vi "PM5000_Harmonics_Results.vi"(8 "error in":errorcluster, 11 "Network Path":string="172.22.26.202") -> (0 "error out":errorcluster, 2 "harmonics out":sgl[](array[numeric]), 3 "Network Path out":string="192.168.169.1")   [LabVIEW 2018]
doc: "Lee la tabla de memoria RealTime_VIF_Power del equipo PowerMonitor 5000, ademas filtra y ordena las variables de interez de la tabla de memoria.\n\nLee las siguientes variables de la tabla RealTime_VIF_Power:\n\n*V1_V2_Volts\n*V2_V3_Volts\n*V3_V1_Volts\n*I1_Amps\n*I2_Amps\n*I3_Amps\n*Frequency_Hz\n*Total_kW\n*Total_kVAR\n*Total_kVA\n*Total_True_PF\n*Total_Disp_PF"
uses:
  <vilib>/ethernetip/ethernetip.llb/EthernetIP SLC500 Read Float.vi
  <vilib>/ethernetip/ethernetip.lvlib
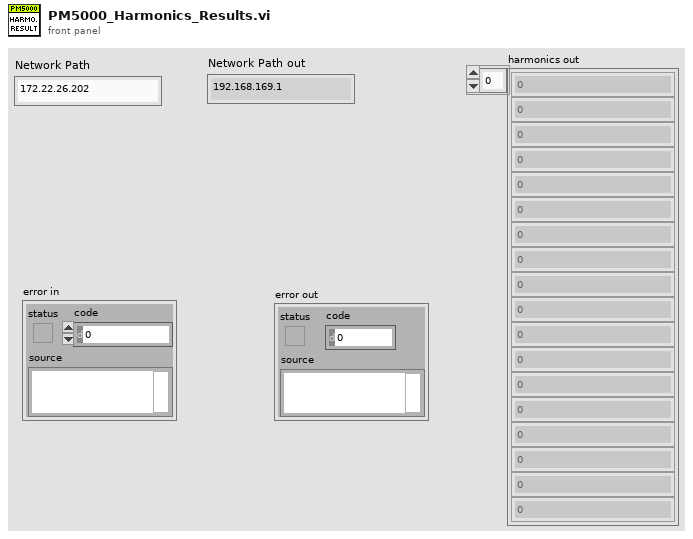
[diagram p1: front panel]
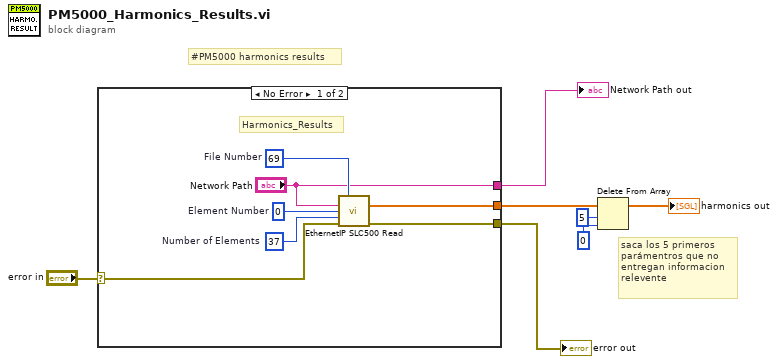
[diagram p0: block diagram]
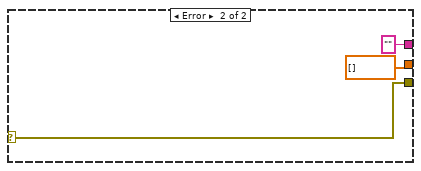
[diagram p2: hidden frame]
diagram:
  # "saca los 5 primeros \nparámentros que no\nentregan informacion\nrelevente"
  # "#PM5000 harmonics results"
  n1 = case shown="No Error" "error in" {
    selector: "error in" -> [w10 w17]
    tunnel: [w11 w17] -> w7
    tunnel: ["Network Path" "" ("Network Path")] -> w5
    tunnel: [w8 sgl[] [] ("Data")] -> w2
    frame No Error {
      w12 = u32 37  # Number of Elements
      w14 = u16 69  # File Number
      w13 = u16 0  # Element Number
      # "Harmonics_Results"
      n2 = call-poly <vilib>:"EthernetIP SLC500 Read.vi"("File Number"=w14, "Network Path"="Network Path", "Element Number"=w13, "Number of Elements"=w12, "error in"=w10) -> ("Data"=w8:sgl[], "error out"=w11:errorcluster)  [unwired: 8 in, 1 out]
    }
    frame Error {
    }
  }
  "error out" <- w7
  "Network Path out" <- w5
  n3 = Delete From Array(array=w2, length=5, index=0) -> (array with subset deleted=→"harmonics out":sgl[])  [unwired: 1 out]
